vi "Neocera Control Panel.vi"(8 "error in (no error)":errorcluster, 11 "Class":refnum<class "Neocera LTC-21.lvclass">) -> (0 "error out":errorcluster, 3 "Neocera LTC-21 out":refnum<class "Neocera LTC-21.lvclass">)   [LabVIEW 2015, in "Neocera LTC-21.lvclass"]
uses:
  Neocera LTC-21.lvclass
  Neocera Front Panel Data.ctl
  Neocera Heater Ranges.ctl
  Neocera Set Point Aproach.ctl
panel:
  in  "Data":T1={"Channels to measure"=[1.0], "Record heater"=FALSE, "Set point"=0.0, "Set Heater Range"=enum."Off", "Control"=FALSE, "Approach"=enum."Instant", "Ramp rate, K/min"=1.0, "Control Channel"=1, "P"=0.0, "I"=0.0, "D"=0.0, "Suspend heater"=FALSE}
  # "300x312"
  # "Temperature Monitor"
  # "Temperature Control"
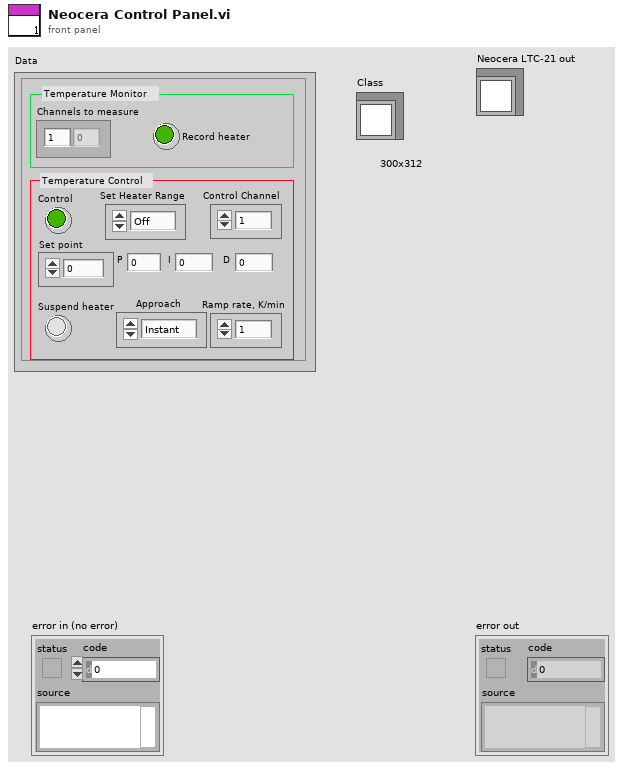
[diagram p1: front panel]
types:
  T1 = typedef "Neocera Front Panel Data.ctl" = cluster{"Channels to measure":dbl[], "Record heater":bool, "Set point":dbl, "Set Heater Range":T2, "Control":bool, "Approach":T3, "Ramp rate, K/min":dbl, "Control Channel":i16, "P":dbl, "I":dbl, "D":dbl, "Suspend heater":bool}
  T2 = typedef "Neocera Heater Ranges.ctl" = enum16{"Off", "0.05W", "0.5W", "5W", "50W"}
  T3 = typedef "Neocera Set Point Aproach.ctl" = enum16{"Instant", "Ramp"}
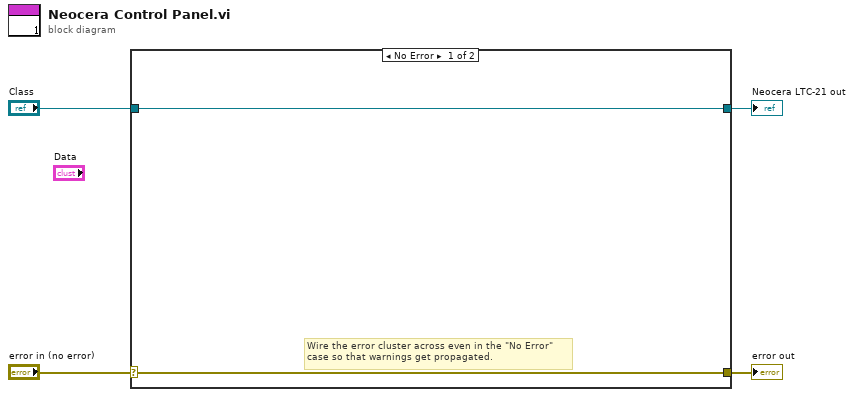
[diagram p0: block diagram]
diagram:
  n1 = case shown="No Error" "error in (no error)" {
    selector: "error in (no error)" -> [w5 w8]
    tunnel: [w5 w8] -> w3
    tunnel: [w6 w7] -> w1
    tunnel: "Class" -> [w6 w7]
    frame No Error {
      # "Wire the error cluster across even in the \"No Error\"\ncase so that warnings get propagated."
    }
    frame Error {
    }
  }
  "error out" <- w3
  "Neocera LTC-21 out" <- w1
